vi "Ocean Optics 2000 4000 Spectrometer DaQ.vi"() -> ()   [LabVIEW 2012]
doc: "Demonstrates continuous waveform measurement. Spectrum is displayed in a waveform graph."
uses:
  Ocean Optics usb 2000 4000/Ocean Optics 2000 4000/Ocean Optics 2000 4000.lvlib
  <vilib>/Utility/file.llb/Write Delimited Spreadsheet (DBL).vi
panel:
  in  "Time For Inner Loop (s)":dbl=2.0 caption="Time Target (s)"
  in  "End Wavelength (< 1040 nm)":dbl format="%#_13g"
  in  "Start Wavelength (> 340 nm)":dbl format="%#_13g"
  in  "Time to Run (s)":dbl format="%#_13g"
  in  "Enable Strobe (Disabled)":bool
  in  "VISA resource name":refnum<visa-resource-name>
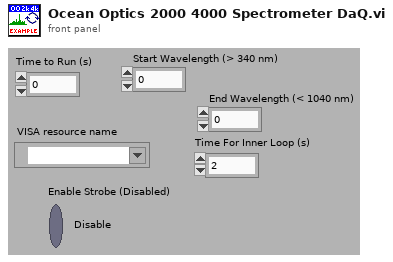
[diagram p1: front panel]
types:
  T1 = cluster{"Wavelength (nm)":dbl[], "Spectrum by Pixel Number":dbl[]}
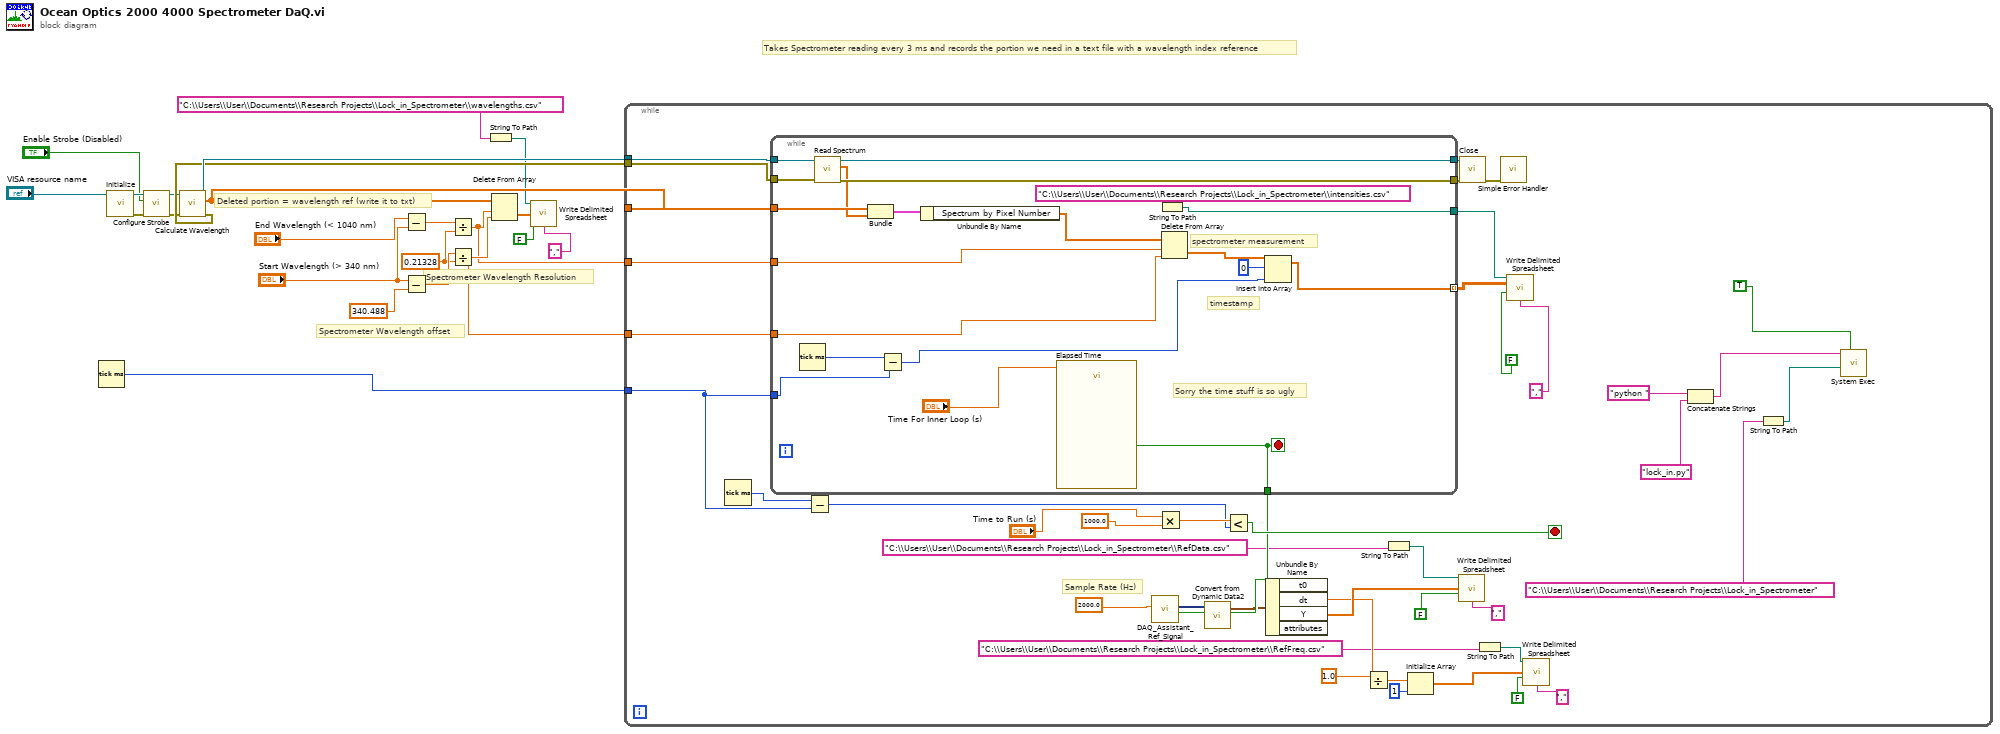
[diagram p0: block diagram]
diagram:
  w7 = 0.21328
  # "Spectrometer Wavelength Resolution"
  # "Spectrometer Wavelength offset"
  # "Takes Spectrometer reading every 3 ms and records the portion we need in a text file with a wavelength index reference"
  # "Deleted portion = wavelength ref (write it to txt)"
  n1 = Tick Count (ms)() -> (millisecond timer value=w5:u32)
  n2 = call "Initialize.vi"("VISA resource name"="VISA resource name") -> ("error out"=w22:errorcluster, "VISA resource name out"=w23:refnum<visa-resource-name>)  [unwired: 2 in, 7 out]
  n3 = call "Configure Strobe.vi"("error in (no error)"=w22, "Enable Strobe (Disabled)"="Enable Strobe (Disabled)", "VISA resource name"=w23) -> ("error out"=w16:errorcluster, "VISA resource name out"=w17:refnum<visa-resource-name>)  [unwired: 7 out]
  n4 = call "Calculate Wavelength.vi"("error in (no error)"=w16, "VISA resource name"=w17) -> ("error out"=w18:errorcluster, "Wavelength (nm)"=w15:dbl[], "VISA resource name out"=w19:refnum<visa-resource-name>)  [unwired: 1 in, 6 out]
  n5 = Subtract(x="End Wavelength (< 1040 nm)", y="Start Wavelength (> 340 nm)") -> (x-y=w8:dbl)
  n6 = Subtract(x="Start Wavelength (> 340 nm)", y=340.488) -> (x-y=w12:dbl)
  n7 = Divide(x=w8, y=w7) -> (x/y=w6:dbl)
  n8 = Divide(x=w12, y=w7) -> (x/y=w11:dbl)
  n9 = String To Path(string="C:\\Users\\User\\Documents\\Research Projects\\Lock_in_Spectrometer\\wavelengths.csv") -> (path=w2:path)
  n10 = Delete From Array(array=w15, length=w6, index=w11) -> (deleted portion=w14:dbl[])  [unwired: 1 out]
  n11 = call-poly <vilib>:"Write Delimited Spreadsheet.vi"("file path (dialog if empty)"=w2, "1D data"=w14, "append to file? (new file:F)"=FALSE, "delimiter (\\t)"=",") -> ()  [unwired: 10 in, 2 out]
  n12 = while {
    tunnel: w19 -> [w63]
    tunnel: w18 -> [w62]
    tunnel: w15 -> [w61]
    tunnel: w11 -> [w60]
    tunnel: w6 -> [w59]
    tunnel: w5 -> [w50]
    stop <- w58 stop-if-true
    # "Sample Rate (Hz)"
    n13 = Tick Count (ms)() -> (millisecond timer value=w51:u32)
    n14 = while {
      tunnel: [w86] -> w66
      tunnel: [w85] -> w65
      tunnel: w61 -> [w84]
      tunnel: w63 -> [w82]
      tunnel: w62 -> [w81]
      tunnel: w59 -> [w78]
      tunnel: w60 -> [w77]
      tunnel: [w68] -> w54
      tunnel: [w74] -> w49 mode=indexing
      tunnel: w50 -> [w72]
      tunnel: [w67] -> w44
      stop <- w67 stop-if-true
      # "Sorry the time stuff is so ugly"
      # "spectrometer measurement"
      # "timestamp"
      n15 = Tick Count (ms)() -> (millisecond timer value=w73:u32)
      n16 = call "Read Spectrum.vi"("error in (no error)"=w81, "VISA resource name"=w82) -> ("error out"=w85:errorcluster, "Spectrum by Pixel Number"=w83:dbl[], "VISA resource name out"=w86:refnum<visa-resource-name>)  [unwired: 6 in, 1 out]
      n17 = Bundle("Wavelength (nm)"=w84, "Spectrum by Pixel Number"=w83) -> (w80:T1)  [unwired: 1 out]
      n18 = Subtract(x=w73, y=w72) -> (x-y=w71:u32)
      n19 = Unbundle By Name(w80) -> ("Spectrum by Pixel Number"=w79:dbl[])
      n20 = call "Elapsed Time"("Time Target (s)"="Time For Inner Loop (s)") -> ("Time has Elapsed"=w67:bool)  [unwired: 11 in, 7 out]
      n21 = String To Path(string="C:\\Users\\User\\Documents\\Research Projects\\Lock_in_Spectrometer\\intensities.csv") -> (path=w68:path)
      n22 = Delete From Array(array=w79, length=w78, index=w77) -> (deleted portion=w76:dbl[])  [unwired: 1 out]
      n23 = Insert Into Array(array=w76, index=0, new element=w71) -> (w74:dbl[])
    }
    n24 = Subtract(x=w51, y=w50) -> (x-y=w48:u32)
    n25 = call "DAQ_Assistant_Ref_Signal.vi"("stop (F)"=w44, "rate"=2000.0) -> ("data 2"=w43:dynamicdata)  [unwired: 9 in]
    n26 = Multiply(x="Time to Run (s)", y=1000.0) -> (x*y=w57:dbl)
    n27 = call "Convert from Dynamic Data2"("Dynamic Data Type"=w43) -> ("Waveform"=w42:waveform(dbl))  [unwired: 3 in]
    n28 = Less?(x=w57, y=w48) -> (x < y?=w58:bool)
    n29 = Unbundle By Name(w42) -> ("dt"=w36:dbl, "Y"=w39:dbl[])  [unwired: 2 out]
    n30 = Divide(x=1.0, y=w36) -> (x/y=w30:dbl)
    n31 = String To Path(string="C:\\Users\\User\\Documents\\Research Projects\\Lock_in_Spectrometer\\RefData.csv") -> (path=w37:path)
    n32 = Initialize Array(w30, 1 ("dimension size")) -> (w28:dbl[])
    n33 = call-poly <vilib>:"Write Delimited Spreadsheet.vi"("file path (dialog if empty)"=w37, "1D data"=w39, "append to file? (new file:F)"=FALSE, "delimiter (\\t)"=",") -> ()  [unwired: 10 in, 2 out]
    n34 = call "Close.vi"("error in (no error)"=w65, "VISA resource name"=w66) -> ("error out"=w64:errorcluster)  [unwired: 9 out]
    n35 = String To Path(string="C:\\Users\\User\\Documents\\Research Projects\\Lock_in_Spectrometer\\RefFreq.csv") -> (path=w32:path)
    n36 = call <vilib>:"Simple Error Handler.vi"("error in (no error)"=w64) -> ()  [unwired: 1 in, 8 out]
    n37 = call-poly <vilib>:"Write Delimited Spreadsheet.vi"("file path (dialog if empty)"=w54, "2D data"=w49, "append to file? (new file:F)"=FALSE, "delimiter (\\t)"=",") -> ()  [unwired: 10 in, 2 out]
    n38 = call-poly <vilib>:"Write Delimited Spreadsheet.vi"("file path (dialog if empty)"=w32, "1D data"=w28, "append to file? (new file:F)"=FALSE, "delimiter (\\t)"=",") -> ()  [unwired: 10 in, 2 out]
    n39 = Concatenate Strings("python " ("string"), "lock_in.py" ("string")) -> (w47:string)
    n40 = String To Path(string="C:\\Users\\User\\Documents\\Research Projects\\Lock_in_Spectrometer") -> (path=w26:path)
    n41 = call <vilib>:"System Exec.vi"("wait until completion? (T)"=TRUE, "working directory"=w26, "command line"=w47) -> ()  [unwired: 5 in, 4 out]
  }
